vi "Build Display Preview.vi"(8 "error in (no error)":errorcluster, 11 "Display Areas":T1(array[cluster])) -> (0 "error out":errorcluster, 3 "Display Preview":picture)   [LabVIEW 2020, in "MacroAssert.lvlib"]
doc: "Outputs a 2D picture representing the orientation of all displays."
uses:
  MacroAssert.lvlib
  <vilib>/Analysis/NI_AALBase.lvlib
  <vilib>/Analysis/baseanly.llb/Mean (DBL).vi
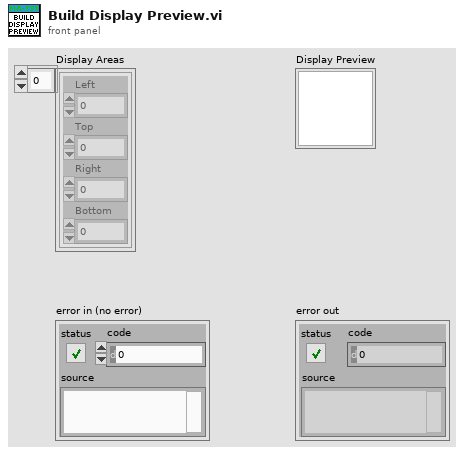
[diagram p1: front panel]
types:
  T1 = cluster{"Left":i32, "Top":i32, "Right":i32, "Bottom":i32}[]
  T2 = cluster{"horizontal":enum16{"left", "center", "right"}, "vertical":enum16{"top", "center", "bottom"}}
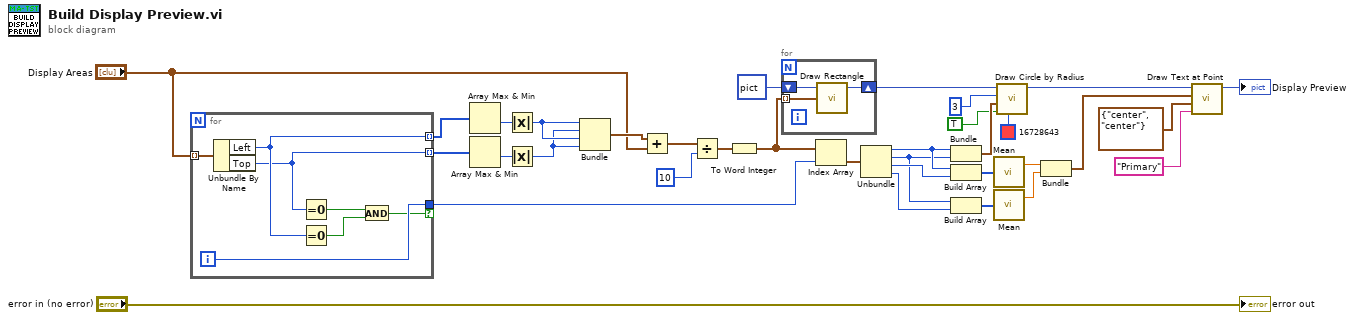
[diagram p0: block diagram]
diagram:
  n1 = for {
    tunnel: [w39] -> w7 mode=indexing
    tunnel: [w38] -> w31 mode=indexing
    tunnel: [w41] -> w21 if=w35
    tunnel: "Display Areas" -> [w40] mode=indexing
    i -> [w41]
    n2 = Unbundle By Name(w40) -> ("Left"=w39:i32, "Top"=w38:i32)
    n3 = Equal To 0?(x=w38) -> (x = 0?=w37:bool)
    n4 = Equal To 0?(x=w39) -> (x = 0?=w36:bool)
    n5 = And(x=w37, y=w36) -> (x .and. y?=w35:bool)
  }
  n6 = Array Max & Min(array=w7) -> (min value=w30:i32)  [unwired: 3 out]
  n7 = Array Max & Min(array=w31) -> (min value=w29:i32)  [unwired: 3 out]
  n8 = Absolute Value(x=w30) -> (abs(x)=w6:i32)
  n9 = Absolute Value(x=w29) -> (abs(x)=w5:i32)
  n10 = Bundle(w6, w5, w6, w5) -> (w4:cluster{i32, i32, i32, i32})  [unwired: 1 in]
  n11 = Add(x=w4, y="Display Areas") -> (x+y=w3:cluster{i32, i32, i32, i32}[])
  n12 = Divide(x=w3, y=10) -> (x/y=w22:cluster{dbl, dbl, dbl, dbl}[])
  n13 = To Word Integer(number=w22) -> (16bit integer=w20:cluster{i16, i16, i16, i16}[])
  n14 = for {
    shift-right: [w43] -> w25
    shift-left: picture data[5B] ("picture") -> [w44]
    tunnel: w20 -> [w42] mode=indexing
    n15 = call <vilib>:"Draw Rectangle.vi"("picture"=w44, "rect"=w42) -> ("new picture"=w43:picture)  [unwired: 7 in]
  }
  n16 = Index Array(array=w20, index=w21) -> (element=w19:cluster{i16, i16, i16, i16})
  n17 = Unbundle(w19) -> (w17:i16, w15:i16, w16:i16, w14:i16)
  n18 = Bundle(w17, w15) -> (w32:cluster{i16, i16})  [unwired: 1 in]
  n19 = Build Array(w17, w16) -> (w13:i16[])
  n20 = Build Array(w15, w14) -> (w12:i16[])
  n21 = call-poly <vilib>:"Mean.vi"("X"=w13) -> ("mean"=w11:dbl)  [unwired: 1 out]
  n22 = call-poly <vilib>:"Mean.vi"("X"=w12) -> ("mean"=w10:dbl)  [unwired: 1 out]
  n23 = call <vilib>:"Draw Circle by Radius.vi"("color(black)"=u32 16728643, "fill?(F)"=TRUE, "pixel center"=w32, "radius"=i16 3, "picture"=w25) -> ("new picture"=w18:picture)  [unwired: 6 in]
  n24 = Bundle("mean"=w11, "mean"=w10) -> (w9:cluster{"mean":dbl, "mean":dbl})  [unwired: 1 in]
  n25 = call <vilib>:"Draw Text at Point.vi"("text"="Primary", "alignment(left, top)"=T2 {"horizontal"=enum."center", "vertical"=enum."center"}, "origin"=w9, "picture"=w18) -> ("new picture"=→"Display Preview":picture)  [unwired: 6 in, 1 out]
  "error out" <- "error in (no error)"
